vi "Opg 2.40 Arrays.vi"() -> ()   [LabVIEW 2022 SP3]
panel:
  in  "Delete?":bool
  in  "Index to delete":i32
  in  "Runs":i32
  out "Array":dbl[](array[numeric])
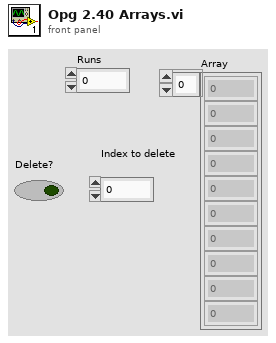
[diagram p1: front panel]
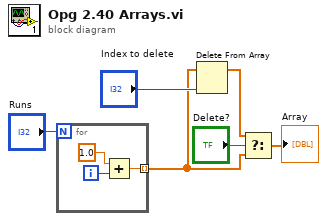
[diagram p0: block diagram]
diagram:
  n1 = for {
    N: "Runs" -> [_]
    tunnel: [w7] -> w1 mode=indexing
    i -> [w8]
    n2 = Add(x=1.0, y=w8) -> (x+y=w7:dbl)
  }
  n3 = Delete From Array(array=w1, index="Index to delete") -> (array with subset deleted=w2:dbl[])  [unwired: 1 in, 1 out]
  n4 = Select(t=w2, s="Delete?", f=w1) -> (s? t:f=→"Array":dbl[])
